vi "Set Current (seq) (SubVI).vi"(10 "字符串":string, 11 "队列输入":refnum<queue>) -> ()   [LabVIEW 2019, in "Take Seq.lvlib"]
uses:
  Take Seq.lvlib
  config.ctl
  lib/QDInstrument.dll
  SubVI.lvlib
panel:
  # "(真是通道1，假是通道2)"
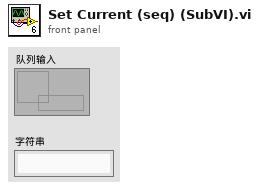
[diagram p1: front panel]
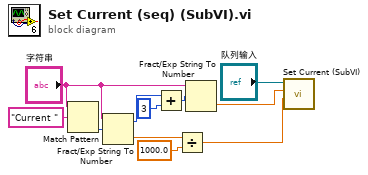
[diagram p0: block diagram]
diagram:
  n1 = Match Pattern(string="字符串", regular expression="Current " ("正则表达式")) -> (offset past match=w10:i32)  [unwired: 1 in, 3 out]
  n2 = Fract/Exp String To Number(string="字符串", offset=w10) -> (offset past number=w8:i32, number=w4:dbl)  [unwired: 2 in]
  n3 = Add(x=w8, y=3) -> (x+y=w9:i32)
  n4 = Divide(x=w4, y=1000.0) -> (x/y=w2:dbl)
  n5 = Fract/Exp String To Number(string="字符串", offset=w9) -> (number=w1:dbl)  [unwired: 2 in, 1 out]
  n6 = call "Set Current (SubVI).vi"("current(A)"=w2, "freq"=w1, "队列输入"="队列输入") -> ()  [unwired: 9 in]
